vi "Run.vi"(8 "error in (no error)":errorcluster, 10 "device address":string, 11 "Engine Simulation Session in":refnum<class "Engine Simulation Session.lvclass">) -> (0 "error out":errorcluster, 3 "Engine Simulation Session out":refnum<class "Engine Simulation Session.lvclass">)   [LabVIEW 2013, in "Engine Simulation Session.lvclass"]
uses:
  Engine Simulation Session.lvclass
  Engine Simulation Session.lvclass/Engine Simulation Session.ctl
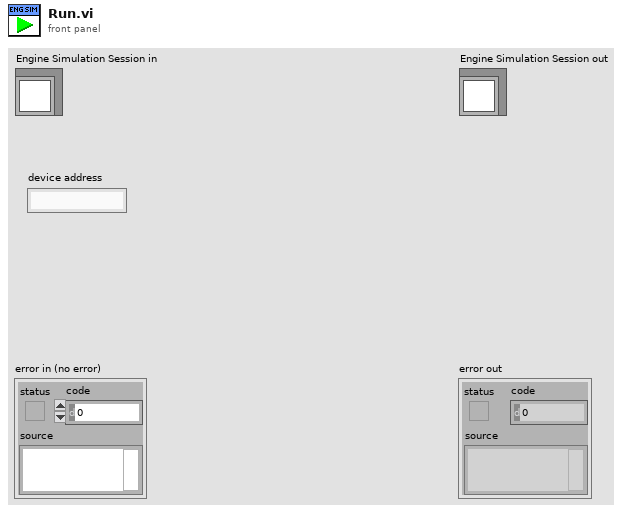
[diagram p1: front panel]
types:
  T1 = typedef "Engine Simulation Session.lvclass/session class private data.ctl" = cluster{"running":bool, "fpga reference":refnum<k20>, "bitfile":path}
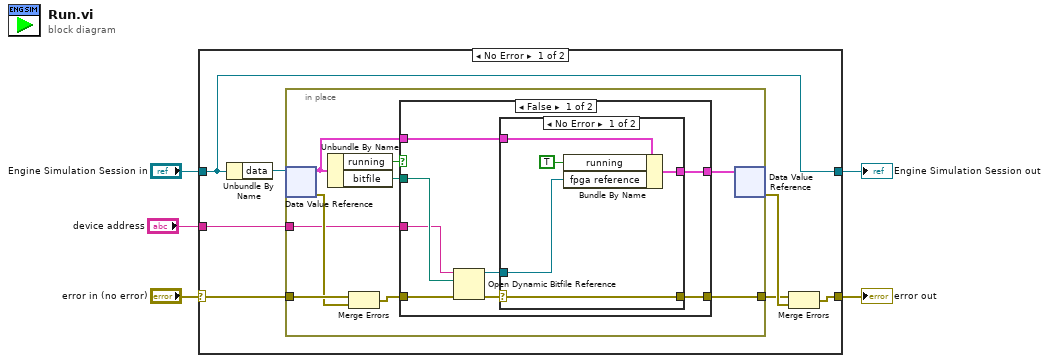
[diagram p0: block diagram]
diagram:
  n1 = case shown="No Error" "error in (no error)" {
    selector: "error in (no error)" -> [w12 w40]
    tunnel: [w6 w40] -> w4
    tunnel: [w10 w39] -> w2
    tunnel: "Engine Simulation Session in" -> [w10 w39]
    tunnel: "device address" -> [w9 _]
    frame No Error {
      n2 = Unbundle By Name(w10) -> ("data"=w11:refnum<data-value>)
      n3 = in-place {
        in-place-border: w12 -> [w21]
        in-place-border: w9 -> [w16]
        in-place-border: [w13] -> w7
        n4 = in-place-dvr #1(w11) -> (w15:T1, w20:errorcluster)
        n5 = Unbundle By Name(w15) -> ("running"=w18:bool, "bitfile"=w17:path)
        n6 = Merge Errors(w21, w20) -> (w19:errorcluster)
        n7 = case shown="False" w18 {
          tunnel: w19 -> [w29 w37]
          tunnel: w17 -> [w28 _]
          tunnel: w16 -> [w27 _]
          tunnel: w15 -> [w26 w38]
          tunnel: [w22 w37] -> w13
          tunnel: [w24 w38] -> w14
          frame False {
            n8 = Open Dynamic Bitfile Reference(0:w27, 1:w28, 3:w29) -> (5:w25:refnum<k20>, 8:w23:errorcluster)  [unwired: 2 in]
            n9 = case shown="No Error" w23 {
              selector: w23 -> [w30 w35]
              tunnel: w26 -> [w34 w36]
              tunnel: w25 -> [w33 _]
              tunnel: [w32 w36] -> w24
              tunnel: [w30 w35] -> w22
              frame No Error {
                n10 = Bundle By Name(cluster=w34, "running"=TRUE, "fpga reference"=w33) -> (w32:T1)
              }
              frame Error {
              }
            }
          }
          frame True {
            # "#todo already running error"
          }
        }
        n11 = in-place-dvr #1(w14) -> (w8:errorcluster)  [unwired: 1 out]
      }
      n12 = Merge Errors(w7, w8) -> (w6:errorcluster)
    }
    frame Error {
    }
  }
  "error out" <- w4
  "Engine Simulation Session out" <- w2
